vi "Msg To.vi"(9 "Event jettl":refnum<class "Event jettl.lvclass">, 10 "Alias":string) -> (3 "Event Create Msg Strategy out":refnum<class "Event Create Msg Strategy.lvclass">)   [LabVIEW 2021, in "jettl.lvlib" / "Event Create.lvlib"]
uses:
  Event Create.lvlib
  Event Create Msg Strategy/Event Create Msg Strategy.lvclass
  Event jettl/Event jettl.lvclass
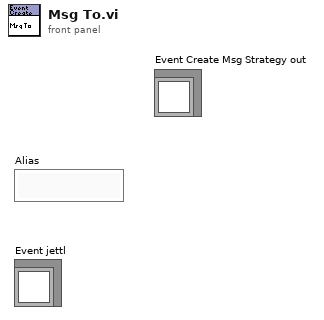
[diagram p1: front panel]
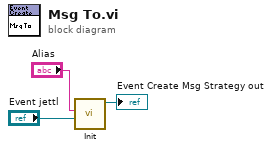
[diagram p0: block diagram]
diagram:
  n1 = call "Init.vi"("Event jettl"="Event jettl", "Alias"="Alias") -> ("Event Create Msg Strategy out"=→"Event Create Msg Strategy out":refnum<class "Event Create Msg Strategy.lvclass">)  [unwired: 9 in]
